vi "Baby Shark Initialization VI.vi"(8 "error in (no error)":errorcluster, 10 "Custom XML":string, 11 "Device Item Ref in":T1 format="%.0x") -> (0 "error out":errorcluster, 3 "Device Item Ref out":T1 format="%.0x")   [LabVIEW 2018, in "Baby Shark Custom Device.lvlib"]
uses:
  Baby Shark Custom Device.lvlib
  <vilib>/NI Veristand/Custom Device API/Custom Device Item Ref.ctl
  <vilib>/NI Veristand/Custom Device API/Custom Device Channel.ctl
  <vilib>/NI Veristand/Custom Device API/Custom Device Channel Type.ctl
  <vilib>/NI Veristand/Custom Device API/Custom Device API.lvlib
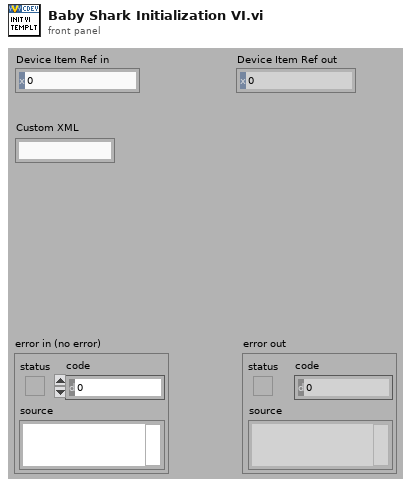
[diagram p1: front panel]
types:
  T1 = typedef "Custom Device API.lvlib/Custom Device Item Ref.ctl" = u64
  T2 = typedef "Custom Device API.lvlib/Custom Device Channel.ctl" = cluster{"Type":T3, "Units":string, "Default Value":dbl, "Faultable":bool, "Scalable":bool}
  T3 = typedef "Custom Device API.lvlib/Custom Device Channel Type.ctl" = enum16{"Input", "Output"}
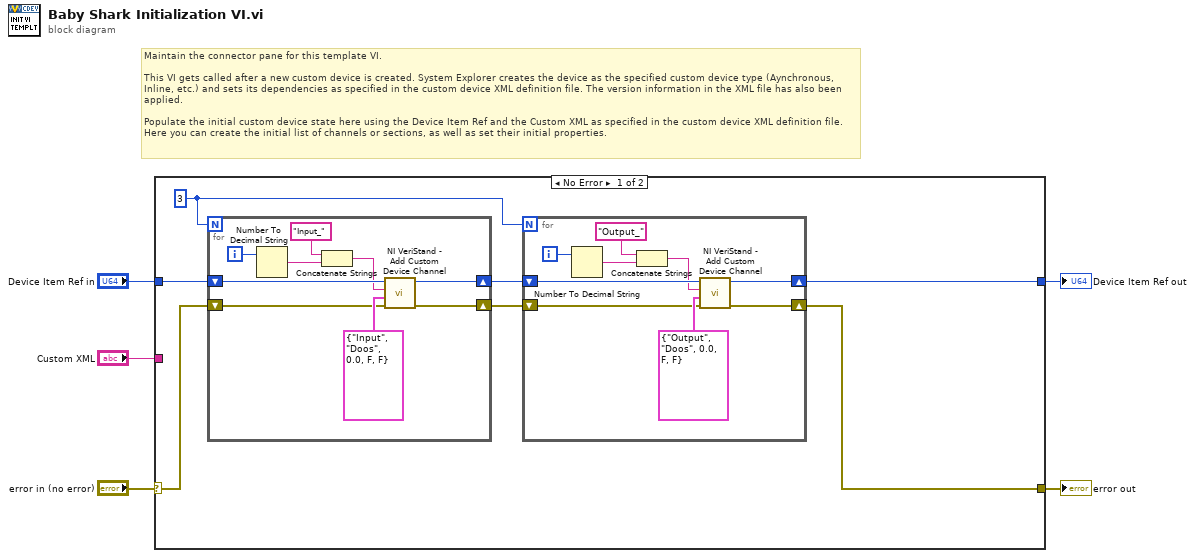
[diagram p0: block diagram]
diagram:
  # "Maintain the connector pane for this template VI.\n\nThis VI gets called after a new custom device is created. System Explorer creates the device as the specified custom device type (Aynchronous, Inline, etc.) and sets its dependencies as specified in the custom device XML definition file. The version information in the XML file has also been applied.\n\nPopulate the initial custom device state here using the Device Item Ref and the Custom XML as specified in the custom device XML definition file. Here you can create the initial list of channels or sections, as well as set their initial properties."
  n1 = case shown="No Error" "error in (no error)" {
    selector: "error in (no error)" -> [w11 w32]
    tunnel: [w6 w32] -> w5
    tunnel: [w7 w31] -> w3
    tunnel: "Device Item Ref in" -> [w12 w31]
    tunnel: "Custom XML" -> [_ _]
    frame No Error {
      w8 = 3
      n2 = for {
        N: w8 -> [_]
        shift-right: [w29] -> w10
        shift-left: w12 -> [w30]
        shift-right: [w22] -> w9
        shift-left: w11 -> [w23]
        i -> [w27]
        n3 = Number To Decimal String(number=w27) -> (decimal integer string=w26:string)  [unwired: 1 in]
        n4 = Concatenate Strings("Input_" ("string"), w26) -> (w24:string)
        n5 = call <vilib>:"NI VeriStand - Add Custom Device Channel.vi"("error in (no error)"=w23, "Channel"=T2 {"Type"=enum."Input", "Units"="Doos", "Default Value"=0.0, "Faultable"=FALSE, "Scalable"=FALSE}, "Channel Name"=w24, "Parent Ref in"=w30) -> ("error out"=w22:errorcluster, "Parent Ref out"=w29:T1)  [unwired: 4 in, 2 out]
      }
      n6 = for {
        N: w8 -> [_]
        shift-right: [w20] -> w7
        shift-left: w10 -> [w21]
        shift-right: [w13] -> w6
        shift-left: w9 -> [w14]
        i -> [w18]
        n7 = Number To Decimal String(number=w18) -> (decimal integer string=w17:string)  [unwired: 1 in]
        n8 = Concatenate Strings("Output_" ("string"), w17) -> (w15:string)
        n9 = call <vilib>:"NI VeriStand - Add Custom Device Channel.vi"("error in (no error)"=w14, "Channel"=T2 {"Type"=enum."Output", "Units"="Doos", "Default Value"=0.0, "Faultable"=FALSE, "Scalable"=FALSE}, "Channel Name"=w15, "Parent Ref in"=w21) -> ("error out"=w13:errorcluster, "Parent Ref out"=w20:T1)  [unwired: 4 in, 2 out]
      }
    }
    frame Error {
    }
  }
  "error out" <- w5
  "Device Item Ref out" <- w3
